vi "cali_interpolation.vi"(7 "降序?":bool, 10 "插值点数":i32, 11 "array R":dbl[](array[numeric])) -> (3 "插值数组":dbl[](array[numeric]))   [LabVIEW 2017]
doc: "本VI的功能是对采集到的calibration image 进行插值。\n为了保证校准图像大小的一致性，用插值点数来规定插多少个点。\n目前的矩阵是一个递减顺序，因为数据索引是从上往下数的。\n也可以选择升序，从最小值开始升。"
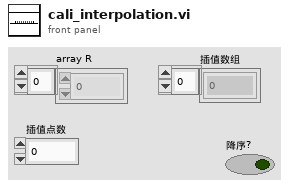
[diagram p1: front panel]
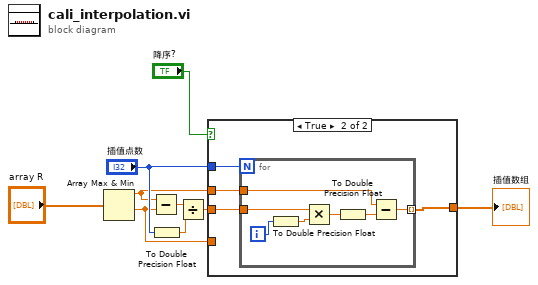
[diagram p0: block diagram]
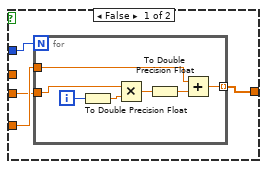
[diagram p2: hidden frame]
diagram:
  n1 = Array Max & Min(array="array R") -> (max value=w3:dbl, min value=w4:dbl)  [unwired: 2 out]
  n2 = Subtract(x=w3, y=w4) -> (x-y=w5:dbl)
  n3 = To Double Precision Float(number="插值点数") -> (double precision float=w8:dbl)
  n4 = Divide(x=w5, y=w8) -> (x/y=w6:dbl)
  n5 = case shown="True" "降序?" {
    tunnel: [w11 w24] -> w9
    tunnel: "插值点数" -> [w10 w23]
    tunnel: w6 -> [w12 w22]
    tunnel: w4 -> [w13 _]
    tunnel: w3 -> [_ w21]
    frame False {
      n6 = for {
        N: w10 -> [_]
        tunnel: w13 -> [w19]
        tunnel: [w16] -> w11 mode=indexing
        tunnel: w12 -> [w14]
        i -> [w20]
        n7 = To Double Precision Float(number=w20) -> (double precision float=w15:dbl)
        n8 = Multiply(x=w14, y=w15) -> (x*y=w18:dbl)
        n9 = To Double Precision Float(number=w18) -> (double precision float=w17:dbl)
        n10 = Add(x=w19, y=w17) -> (x+y=w16:dbl)
      }
    }
    frame True {
      n11 = for {
        N: w23 -> [_]
        tunnel: w21 -> [w30]
        tunnel: [w27] -> w24 mode=indexing
        tunnel: w22 -> [w25]
        i -> [w31]
        n12 = To Double Precision Float(number=w31) -> (double precision float=w26:dbl)
        n13 = Multiply(x=w25, y=w26) -> (x*y=w29:dbl)
        n14 = To Double Precision Float(number=w29) -> (double precision float=w28:dbl)
        n15 = Subtract(x=w30, y=w28) -> (x-y=w27:dbl)
      }
    }
  }
  "插值数组" <- w9
